vi "Leap Swipe Gesture.vi"() -> ()   [LabVIEW 2014, in "LMH-Leap.lvlib"]
doc: "This example demonstrates how to read the vector of a swipe gesture using the Leap Motion Controller."
uses:
  vi.lib/MakerHub/Leap/LMH-Leap.lvlib
  vi.lib/MakerHub/Leap/Public/Gestures/Swipe/Instance VIs/Read 1 Swipe Vector.vi
panel:
  out "Swipe Vector":cluster{"X":sgl, "Y":sgl, "Z":sgl}
  out "X Z Swipe Vector":T1(graph)
  in  "Stop Button":bool
  # "Leap Swipe Gesture Example\n\nThis example demonstrates how to read the vector of a swipe gesture using the Leap Motion Controller.\n\nInstructions\n1. Connect the Leap Motion Controller to the host computer.\n2. Click the Run Arrow.\n3. Make a swipe gesture above the Leap and notice the swipe vector indicated on the graph below."
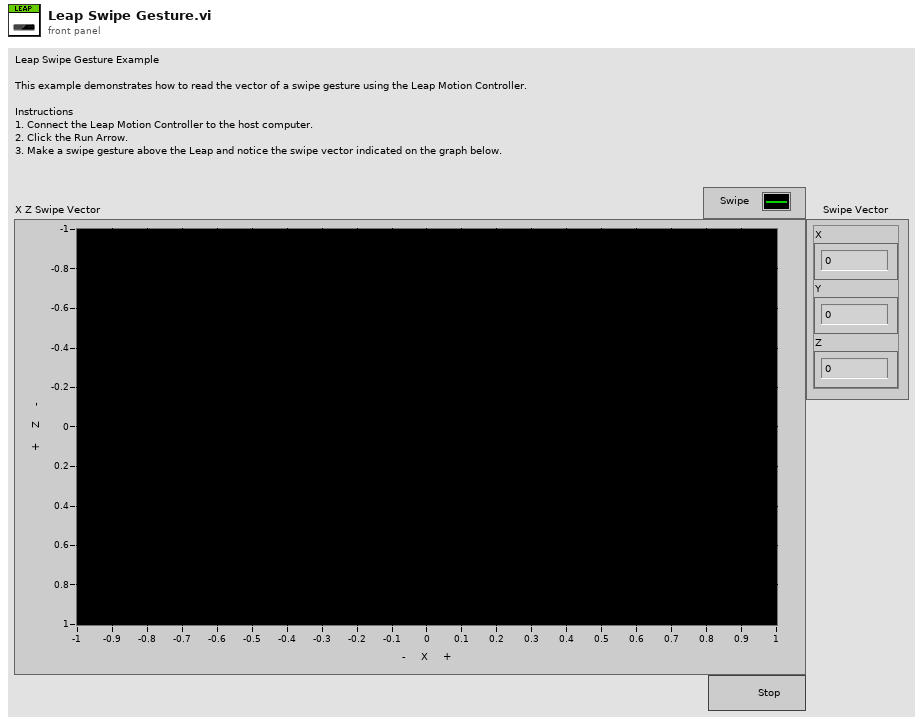
[diagram p1: front panel]
types:
  T1 = cluster{"Numeric Control":sgl, "Numeric Control":dbl}[]
  T2 = typedef "LMH-Leap.lvlib/Leap Handle.ctl" = cluster{"LeapCSharp":refnum<k24>}
  T3 = typedef "LMH-Leap.lvlib/Gesture State.ctl" = enum16{"Invalid", "Start", "Update", "Stop"}
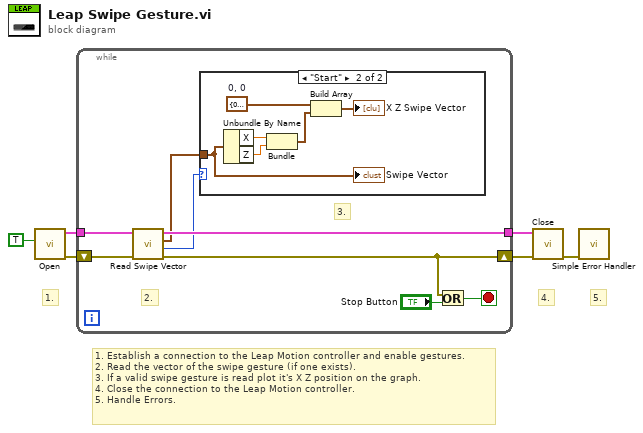
[diagram p0: block diagram]
diagram:
  # "1. Establish a connection to the Leap Motion controller and enable gestures.\n2. Read the vector of the swipe gesture (if one exists).\n3. If a valid swipe gesture is read plot it's X Z position on the graph.\n4. Close the connection to the Leap Motion controller.\n5. Handle Errors."
  # "5."
  # "4."
  # "1."
  n1 = call "Open.vi"("Enable Gestures? (T)"=TRUE) -> ("Error Out"=w4:errorcluster, "Leap Handle"=w6:T2)  [unwired: 9 in]
  n2 = while {
    tunnel: w6 -> [w12]
    shift-right: [w10] -> w5
    shift-left: w4 -> [w9]
    tunnel: [w11] -> w2
    stop <- w14 stop-if-true
    # "3."
    # "2."
    n3 = call-poly "Read Swipe Vector.vi"("Error In"=w9, "Leap Handle"=w12) -> ("Error Out"=w10:errorcluster, "Gesture State"=w7:T3, "Swipe Vector"=w8:cluster{"X":sgl, "Y":sgl, "Z":sgl}, "Leap Handle"=w11:T2)  [unwired: 6 in]
    n4 = case shown="\"Start\"" w7 {
      tunnel: w8 -> [_ w15]
      frame "Invalid", Default {
      }
      frame "Start" {
        w20 = cluster{"Numeric Control":sgl, dbl} {"Numeric Control"=0.0, 0.0}  # 0, 0
        n5 = Unbundle By Name(w15) -> ("X"=w18:sgl, "Z"=w17:sgl)
        n6 = Bundle("X"=w18, "Z"=w17) -> (w16:cluster{"X":sgl, "Z":sgl})  [unwired: 1 in]
        n7 = Build Array(w20, w16) -> (→"X Z Swipe Vector":cluster{"X":sgl, "Z":dbl}[])
        "Swipe Vector" <- w15
      }
    }
    n8 = Or(x=w10, y="Stop Button") -> (x .or. y?=w14:bool)
  }
  n9 = call "Close.vi"("Error In"=w5, "Leap Handle"=w2) -> ("Error Out"=w1:errorcluster)  [unwired: 9 in]
  n10 = call <vilib>:"Simple Error Handler.vi"("error in (no error)"=w1) -> ()  [unwired: 4 in, 5 out]
